vi "Burning CloseQueue.vi"(8 "error in 3":errorcluster, 9 "error in 2":errorcluster, 10 "error in":errorcluster, 11 "queue":refnum<queue>) -> (0 "error out":errorcluster)   [LabVIEW 2022 SP3]
uses:
  Type Def/Burning States.ctl
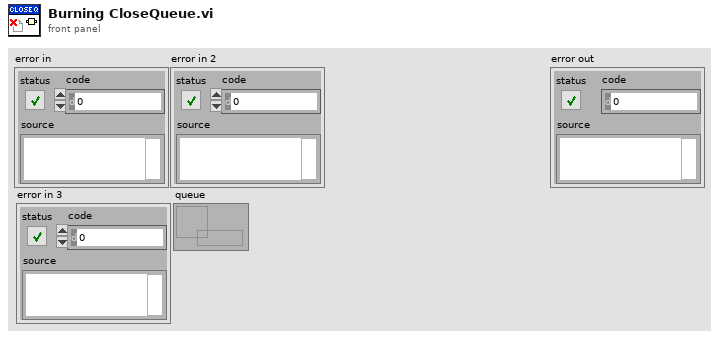
[diagram p1: front panel]
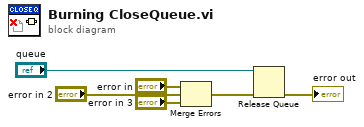
[diagram p0: block diagram]
diagram:
  n1 = Merge Errors("error in", "error in 2", "error in 3") -> (w6:errorcluster)
  n2 = Release Queue(queue="queue", error in (no error)=w6) -> (error out=→"error out":errorcluster)  [unwired: 1 in, 2 out]
